vi "uActor.vi"(8 "error in (no error)":errorcluster, 11 "uActor in":refnum<class "uActor.lvclass">) -> (0 "error out":errorcluster, 3 "uActor out":refnum<class "uActor.lvclass">)   [LabVIEW 2023, in "uLib.lvlib" / "uActor.lvclass"]
doc: "This is the mainasynchronously-called VI that runs as an actor."
uses:
  uActor.lvclass
  uActor.lvclass/uActor.ctl
  uTransport/uTransport_uActor/uTransport_uActor.lvclass/uTransport_uActor.ctl
  uData/uData/uData.lvclass
  uMsg/uMsg/uMsg.lvclass/uMsg.ctl
  uData/uData/uData.lvclass/uData.ctl
  uData/uData/Combine Tags.vi
  uTransport/uTransport/uTransport_SendMsg.vi
  uActor_CMDs_Prefix.vi
  uActor_SendMsg.vi
  uData/uData/Set Tag.vi
  uMsg/uMsg/uMsg Create.vi
  uActor_SimpleSend.vi
  uMsg/uMsg/uMsg Update Timestamp.vi
  uTransport/uTransport_uActor/uTransport_uActor_SendMsg.vi
  uData/uData/Condition Tag Name.vi
  uData/uData/Blank Key Reserved String.vi
  uTransport/uTransport/uTransport.lvclass
  uMsg/uMsg/uMsg.lvclass
  uTransport/uTransport_uActor/uTransport_uActor.lvclass
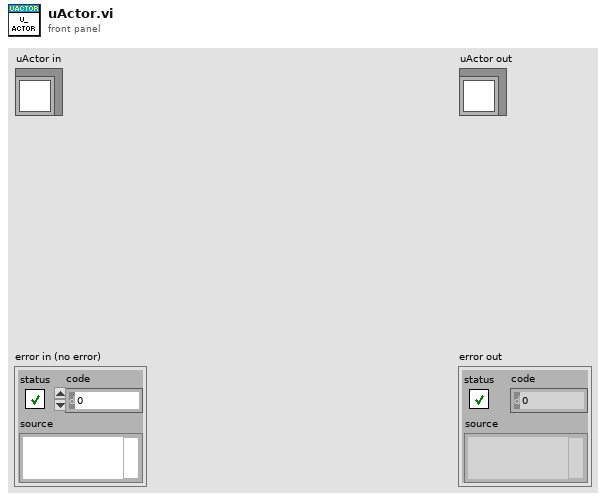
[diagram p1: front panel]
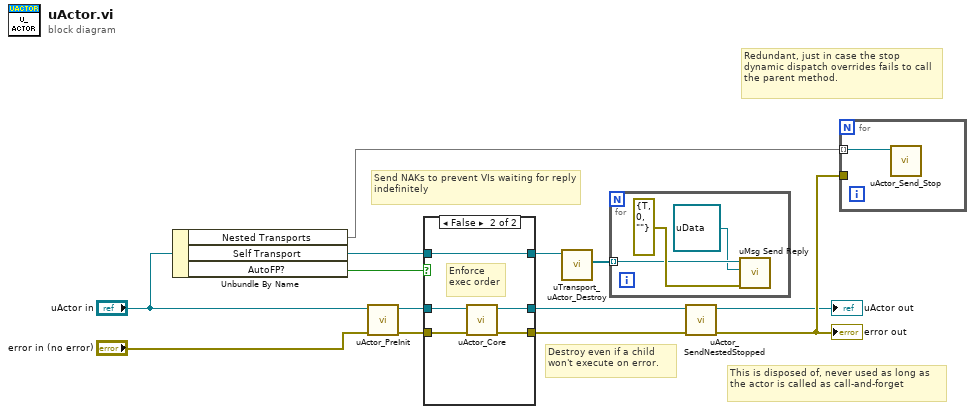
[diagram p0: block diagram]
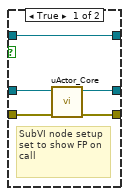
[diagram p2: hidden frame]
diagram:
  # "Destroy even if a child won't execute on error."
  # "Redundant, just in case the stop dynamic dispatch overrides fails to call the parent method."
  # "This is disposed of, never used as long as the actor is called as call-and-forget"
  # "Send NAKs to prevent VIs waiting for reply indefinitely"
  n1 = Unbundle By Name("uActor in") -> ("Nested Transports"=w10:set{refnum<class "uTransport_uActor.lvclass">}, "Self Transport"=w6:refnum<class "uTransport_uActor.lvclass">, "AutoFP?"=w13:bool)
  n2 = call-dynamic "uActor_PreInit.vi"("error in (no error)"="error in (no error)", "uActor in"="uActor in") -> ("error out"=w4:errorcluster, "uActor out"=w2:refnum<class "uActor.lvclass">)  [unwired: 8 in]
  n3 = case shown="False" w13 {
    tunnel: w2 -> [w18 w23]
    tunnel: [w17 w22] -> w7
    tunnel: w4 -> [w16 w21]
    tunnel: [w15 w20] -> w11
    tunnel: w6 -> [w14 w19]
    tunnel: [w14 w19] -> w5
    frame True {
      # "SubVI node setup set to show FP on call"
      n4 = call-dynamic "uActor_Core.vi"("error in (no error)"=w16, "uActor in"=w18) -> ("error out"=w17:errorcluster, "uActor out"=w15:refnum<class "uActor.lvclass">)  [unwired: 8 in]
    }
    frame False {
      # "Enforce exec order"
      n5 = call-dynamic "uActor_Core.vi"("error in (no error)"=w21, "uActor in"=w23) -> ("error out"=w22:errorcluster, "uActor out"=w20:refnum<class "uActor.lvclass">)  [unwired: 8 in]
    }
  }
  n6 = call "uTransport_uActor_Destroy.vi"("uTransport_uActor in"=w5) -> ("remaining elements"=w12:refnum<class "uMsg.lvclass">[])  [unwired: 9 in, 1 out]
  n7 = for {
    tunnel: w12 -> [w25] mode=indexing
    n8 = call "uMsg Send Reply.vi"("error in (no error)"=errorcluster {"status"=TRUE, "code"=0, "source"=""}, "Reply Data"=refnum<class "uData.lvclass"> refnum ("Reply"), "Original Msg"=w25) -> ()  [unwired: 8 in, 1 out]
  }
  n9 = call "uActor_SendNestedStopped.vi"("error in (no error)"=w7, "uActor Last State"=w11) -> ("error out"=w9:errorcluster, "uActor out"=→"uActor out":refnum<class "uActor.lvclass">)  [unwired: 8 in]
  "error out" <- w9
  n10 = for {
    tunnel: w10 -> [w27] mode=indexing
    tunnel: w9 -> [_]
    n11 = call "uActor_Send_Stop.vi"("uActor Transport"=w27) -> ()  [unwired: 10 in, 1 out]
  }
